vi "log_smoothing.vi"(5 "Delay (sec)":sgl format="%#_3p", 6 "N points":u32, 7 "Phase offset (deg)":sgl, 9 "Y":cdb[][](array[numeric]) format="%#_3g", 10 "Frequency range":cluster{"Min":dbl, "Max":dbl}={"Min"=0.0, "Max"=inf} {"Max" format="%#_3p"; "Min" format="%#_3p"}, 11 "Frequency resolution (Hz)":dbl) -> (1 "Y out":cdb[][](array[numeric]) format="%#_3g", 3 "X out":dbl[](array[numeric]))   [LabVIEW 2011]
uses:
  <vilib>/Analysis/1siggen.llb/Ramp Pattern by Samples.vi
  <vilib>/Analysis/NI_AALBase.lvlib
panel:
  # "Smooth some complex spectra by averaging across N logarithmically spaced bins.  The input is as from FFT, with DC component in index 0, and regular spaced frequency bins, with the specified resolution.  The DC component is dropped from the result because it is meaningless to average it in with non-DC responses.  The X values are the result bin center (geometric mean of component frequencies.)"
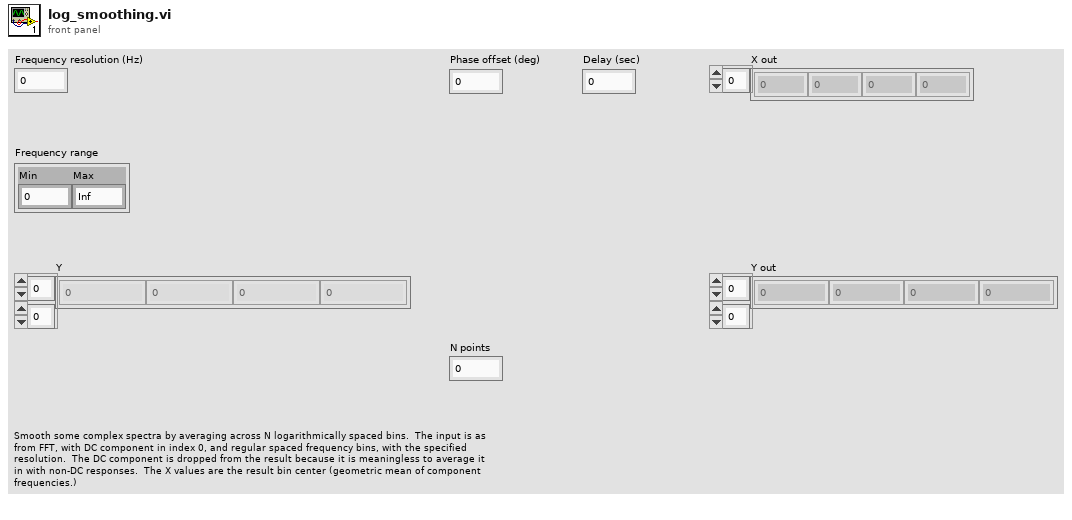
[diagram p1: front panel]
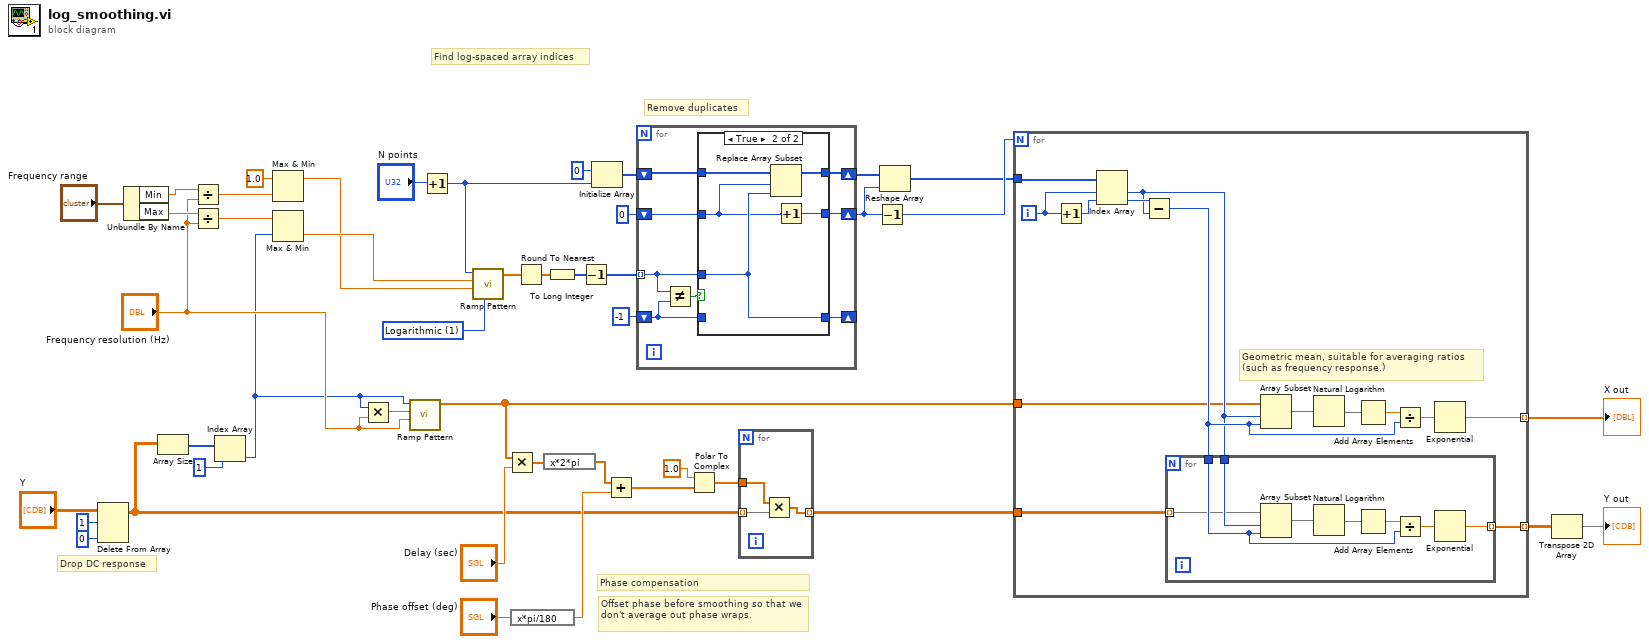
[diagram p0: block diagram]
diagram:
  w45 = u16 1 items=["Linear", "Logarithmic"] ("type")
  # "Offset phase before smoothing so that we don't average out phase wraps."
  # "Phase compensation"
  # "Drop DC response"
  # "Find log-spaced array indices"
  # "Remove duplicates"
  n1 = Delete From Array(array="Y", length=1, index (col)=0 ("disabled index (col)")) -> (array with subset deleted=w6:cdb[][])  [unwired: 1 in, 1 out]
  n2 = Unbundle By Name("Frequency range") -> ("Min"=w22:dbl, "Max"=w21:dbl)
  n3 = Array Size(array=w6) -> (size(s)=w28:i32[])
  n4 = Divide(x=w22, y="Frequency resolution (Hz)") -> (x/y=w16:dbl)
  n5 = Divide(x=w21, y="Frequency resolution (Hz)") -> (x/y=w19:dbl)
  n6 = Index Array(array=w28, index=1) -> (element=w18:i32)
  n7 = Max & Min(x=1.0, y=w16) -> (max(x,y)=w14:dbl)  [unwired: 1 out]
  n8 = Max & Min(x=w19, y=w18) -> (min(x,y)=w17:dbl)  [unwired: 1 out]
  n9 = Multiply(x=w18, y="Frequency resolution (Hz)") -> (x*y=w29:dbl)
  n10 = call-poly <vilib>:"Ramp Pattern.vi"("start"="Frequency resolution (Hz)", "end"=w29, "samples"=w18) -> ("Ramp Pattern"=w9:dbl[])  [unwired: 7 in, 1 out]
  n11 = Increment(x="N points") -> (x+1=w34:u32)
  n12 = call-poly <vilib>:"Ramp Pattern.vi"("type"=w45, "start"=w14, "end"=w17, "samples"=w34) -> ("Ramp Pattern"=w44:dbl[])  [unwired: 6 in, 1 out]
  n13 = Multiply(x=w9, y="Delay (sec)") -> (x*y=w3:dbl[])
  n14 = expression code="x*pi/180"("Phase offset (deg)") -> (w7:sgl)
  n15 = Round To Nearest(number=w44) -> (nearest integer value=w43:dbl[])
  n16 = expression code="x*2*pi"(w3) -> (w2:dbl[])
  n17 = To Long Integer(number=w43) -> (32bit integer=w13:i32[])
  n18 = Decrement(x=w13) -> (x-1=w12:i32[])
  n19 = Initialize Array(0, w34) -> (w39:i32[])
  n20 = Add(x=w2, y=w7) -> (x+y=w1:dbl[])
  n21 = for {
    tunnel: w12 -> [w52] mode=indexing
    shift-right: [w47] -> _
    shift-left: -1 -> [w46]
    shift-right: [w48] -> w36
    shift-left: 0 -> [w49]
    shift-right: [w50] -> w38
    shift-left: w39 -> [w51]
    n22 = Not Equal?(x=w52, y=w46) -> (x != y?=w53:bool)
    n23 = case shown="True" w53 {
      tunnel: w52 -> [_ w59]
      tunnel: w51 -> [w56 w61]
      tunnel: [w56 w60] -> w50
      tunnel: w49 -> [w55 w57]
      tunnel: [w55 w58] -> w48
      tunnel: [w54 w59] -> w47
      tunnel: w46 -> [w54 _]
      frame False {
      }
      frame True {
        n24 = Replace Array Subset(array=w61, new element=w59, index=w57) -> (w60:i32[])
        n25 = Increment(x=w57) -> (x+1=w58:i32)
      }
    }
  }
  n26 = Polar To Complex(1:w1, 2:sgl 1.0 ("r")) -> (0:w5:cdb[])
  n27 = for {
    tunnel: w6 -> [w64] mode=indexing
    tunnel: w5 -> [w63]
    tunnel: [w62] -> w4 mode=indexing
    n28 = Multiply(x=w63, y=w64) -> (x*y=w62:cdb[])
  }
  n29 = Decrement(x=w36) -> (x-1=w37:i32)
  n30 = Reshape Array(w38, w36) -> (w33:i32[])
  n31 = for {
    N: w37 -> [_]
    tunnel: w33 -> [w78]
    tunnel: [w71] -> w31 mode=indexing
    tunnel: w4 -> [w68]
    tunnel: [w67] -> w32 mode=indexing
    tunnel: w9 -> [w66]
    i -> [w77]
    # "Geometric mean, suitable for averaging ratios\n(such as frequency response.)"
    n32 = Increment(x=w77) -> (x+1=w76:i32)
    n33 = Index Array(array=w78, index #1=w77, index #2=w76) -> (element #1=w69:i32, element #2=w75:i32)
    n34 = Subtract(x=w75, y=w69) -> (x-y=w70:i32)
    n35 = for {
      tunnel: w70 -> [w82]
      tunnel: w69 -> [w81]
      tunnel: w68 -> [w80] mode=indexing
      tunnel: [w79] -> w67 mode=indexing
      n36 = Array Subset(array=w80, index=w81, length=w82) -> (w83:cdb[])
      n37 = Natural Logarithm(1:w83) -> (0:w84:cdb[])
      n38 = Add Array Elements(numeric array=w84) -> (sum=w85:cdb)
      n39 = Divide(x=w85, y=w82) -> (x/y=w86:cdb)
      n40 = Exponential(1:w86) -> (0:w79:cdb)
    }
    n41 = Array Subset(array=w66, index=w69, length=w70) -> (w65:dbl[])
    n42 = Natural Logarithm(1:w65) -> (0:w74:dbl[])
    n43 = Add Array Elements(numeric array=w74) -> (sum=w73:dbl)
    n44 = Divide(x=w73, y=w70) -> (x/y=w72:dbl)
    n45 = Exponential(1:w72) -> (0:w71:dbl)
  }
  "X out" <- w31
  n46 = Transpose 2D Array(2D array=w32) -> (transposed array=→"Y out":cdb[][])
